vi "Configure Wavelength.vi"(7 "turret index (0)":u8, 8 "error in (no error)":errorcluster, 9 "reset (false)":bool, 10 "wavelength, nm":dbl, 11 "SOL MS in":refnum<class "PL SOL Instruments MS.lvclass">) -> (0 "error out":errorcluster, 1 "dispersion, nm/mm":dbl, 2 "wavelength, nm":dbl, 3 "SOL MS out":refnum<class "PL SOL Instruments MS.lvclass">)   [LabVIEW 2015, in "PL SOL Instruments MS.lvclass"]
doc: "Configures wavelength."
uses:
  PL SOL Instruments MS.lvclass
  PL SOL Instruments MS.lvclass/PL SOL Instruments MS.ctl
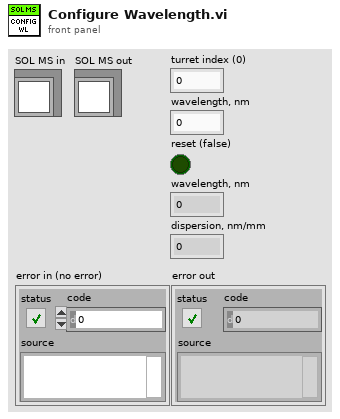
[diagram p1: front panel]
types:
  T1 = cluster{"name":string, "step timeout, ms":u32, "reset timeout, ms":u32, "gratings":cluster{"name":string, "step timeout, ms":u32, "reset timeout, ms":u32, "turret position":i32, "reset position":i32, "max position":i32, "backlash distance":i32, "step size, rad":dbl, "groove density, g/mm":dbl, "theta2, rad":dbl, "blaze wavelength, nm":dbl, "focal length, cm":dbl, "manual change":bool, "manual change position":i32}[], "current grating":cluster{"index":u8, "position":i32}}[]
  T2 = cluster{"name":string, "step timeout, ms":u32, "reset timeout, ms":u32, "gratings":cluster{"name":string, "step timeout, ms":u32, "reset timeout, ms":u32, "turret position":i32, "reset position":i32, "max position":i32, "backlash distance":i32, "step size, rad":dbl, "groove density, g/mm":dbl, "theta2, rad":dbl, "blaze wavelength, nm":dbl, "focal length, cm":dbl, "manual change":bool, "manual change position":i32}[], "current grating":cluster{"index":u8, "position":i32}}
  T3 = cluster{"name":string, "step timeout, ms":u32, "reset timeout, ms":u32, "turret position":i32, "reset position":i32, "max position":i32, "backlash distance":i32, "step size, rad":dbl, "groove density, g/mm":dbl, "theta2, rad":dbl, "blaze wavelength, nm":dbl, "focal length, cm":dbl, "manual change":bool, "manual change position":i32}[]
  T4 = cluster{"name":string, "step timeout, ms":u32, "reset timeout, ms":u32, "turret position":i32, "reset position":i32, "max position":i32, "backlash distance":i32, "step size, rad":dbl, "groove density, g/mm":dbl, "theta2, rad":dbl, "blaze wavelength, nm":dbl, "focal length, cm":dbl, "manual change":bool, "manual change position":i32}
  T5 = cluster{"turrets":cluster{"current grating index":u8, "wavelength, nm":dbl, "dispersion, nm/mm":dbl}[], "shutters":cluster{"is open":bool}[], "mirrors":cluster{"current position index":u8}[], "slits":cluster{"width, um":dbl}[]}
  T6 = cluster{"current grating index":u8, "wavelength, nm":dbl, "dispersion, nm/mm":dbl}[]
  T7 = cluster{"current grating index":u8, "wavelength, nm":dbl, "dispersion, nm/mm":dbl}
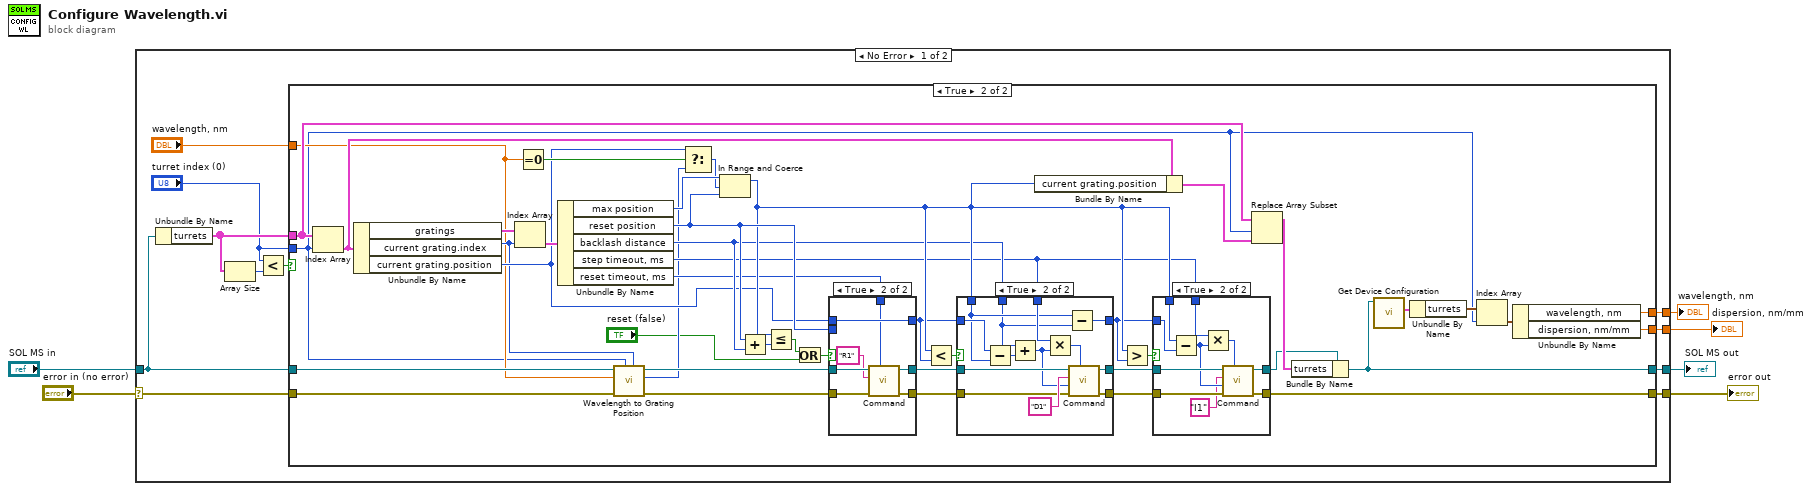
[diagram p0: block diagram]
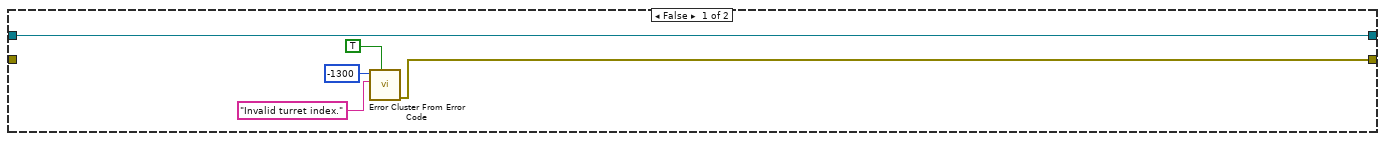
[diagram p2: hidden frame]
diagram:
  n1 = case shown="No Error" "error in (no error)" {
    selector: "error in (no error)" -> [w11 w105]
    tunnel: "SOL MS in" -> [w15 w104]
    tunnel: [w9 _] -> w5
    tunnel: [w8 _] -> w4
    tunnel: [w10 w105] -> w3
    tunnel: [w7 w104] -> w1
    frame No Error {
      n2 = Unbundle By Name(w15) -> ("turrets"=w17:T1)
      n3 = Array Size(array=w17) -> (size(s)=w14:i32)
      n4 = Less?(x="turret index (0)", y=w14) -> (x < y?=w12:bool)
      n5 = case shown="True" w12 {
        tunnel: w11 -> [_ w51]
        tunnel: w15 -> [w22 w49]
        tunnel: [w22 w41] -> w7
        tunnel: [w18 w61] -> w10
        tunnel: w17 -> [_ w59]
        tunnel: "wavelength, nm" -> [_ w47]
        tunnel: "turret index (0)" -> [_ w38]
        tunnel: [_ w40] -> w9
        tunnel: [_ w39] -> w8
        frame False {
          n6 = call <vilib>:"Error Cluster From Error Code.vi"("show call chain? (False)"=TRUE, "error message (\"\")"="Invalid turret index." ("error message (\"\")"), "error code (0)"=-1300) -> ("error out"=w18:errorcluster)  [unwired: 6 in]
        }
        frame True {
          n7 = Index Array(array=w59, index=w38) -> (element=w56:T2)
          n8 = Unbundle By Name(w56) -> ("gratings"=w58:T3, "current grating.index"=w48:u8, "current grating.position"=w53:i32)
          n9 = Index Array(array=w58, index=w48) -> (element=w57:T4)
          n10 = Equal To 0?(x=w47) -> (x = 0?=w54:bool)
          n11 = Unbundle By Name(w57) -> ("max position"=w65:i32, "reset position"=w64:i32, "backlash distance"=w62:i32, "step timeout, ms"=w60:u32, "reset timeout, ms"=w55:u32)
          n12 = call "Wavelength to Grating Position.vi"("grating index (0)"=w48, "turret index (0)"=w38, "error in (no error)"=w51, "wavelength, nm"=w47, "SOL MS in"=w49) -> ("error out"=w45:errorcluster, "grating position"=w46:i32, "SOL MS out"=w50:refnum<class "PL SOL Instruments MS.lvclass">)  [unwired: 4 in]
          n13 = Select(t=w53, s=w54, f=w46) -> (s? t:f=w52:i32)
          n14 = In Range and Coerce(upper limit=w65, x=w52, lower limit=w64) -> (coerced(x)=w63:i32)  [unwired: 1 out]
          n15 = Add(x=w64, y=w62) -> (x+y=w35:i32)
          n16 = Less Or Equal?(x=w63, y=w35) -> (x <= y?=w34:bool)
          n17 = Or(x=w34, y="reset (false)") -> (x .or. y?=w36:bool)
          n18 = case shown="True" w36 {
            tunnel: w50 -> [w96 w99]
            tunnel: w45 -> [w95 w100]
            tunnel: [w95 w101] -> w31
            tunnel: [w96 w102] -> w32
            tunnel: w53 -> [w94 _]
            tunnel: [w94 w103] -> w30
            tunnel: w64 -> [_ w103]
            tunnel: w55 -> [_ w97]
            frame False {
            }
            frame True {
              n19 = call "Command.vi"("additional timeout, ms (0)"=w97, "error in (no error)"=w100, "command"="R1", "SOL MS in"=w99) -> ("error out"=w101:errorcluster, "SOL MS out"=w102:refnum<class "PL SOL Instruments MS.lvclass">)  [unwired: 6 in]
            }
          }
          n20 = Less?(x=w63, y=w30) -> (x < y?=w33:bool)
          n21 = case shown="True" w33 {
            tunnel: w32 -> [w80 w87]
            tunnel: w31 -> [w79 w81]
            tunnel: [w79 w84] -> w29
            tunnel: [w80 w85] -> w28
            tunnel: w30 -> [w78 w91]
            tunnel: [w78 w90] -> w26
            tunnel: w63 -> [_ w89]
            tunnel: w62 -> [_ w88]
            tunnel: w60 -> [_ w92]
            frame False {
            }
            frame True {
              n22 = Subtract(x=w91, y=w89) -> (x-y=w93:i32)
              n23 = Add(x=w88, y=w93) -> (x+y=w82:i32)
              n24 = Multiply(x=w92, y=w82) -> (x*y=w86:u32)
              n25 = Subtract(x=w89, y=w88) -> (x-y=w90:i32)
              n26 = call "Command.vi"("additional timeout, ms (0)"=w86, "error in (no error)"=w81, "data"=w82, "command"="D1", "SOL MS in"=w87) -> ("error out"=w84:errorcluster, "SOL MS out"=w85:refnum<class "PL SOL Instruments MS.lvclass">)  [unwired: 5 in]
            }
          }
          n27 = Bundle By Name(cluster=w56, "current grating.position"=w63) -> (w25:T2)
          n28 = Greater?(x=w63, y=w26) -> (0:w27:bool)
          n29 = case shown="True" w27 {
            tunnel: w28 -> [w67 w73]
            tunnel: w29 -> [w66 w72]
            tunnel: [w66 w69] -> w61
            tunnel: [w67 w68] -> w23
            tunnel: w26 -> [_ w76]
            tunnel: w63 -> [_ w75]
            tunnel: w60 -> [_ w77]
            frame False {
            }
            frame True {
              n30 = Subtract(x=w75, y=w76) -> (x-y=w71:i32)
              n31 = Multiply(x=w77, y=w71) -> (x*y=w74:u32)
              n32 = call "Command.vi"("additional timeout, ms (0)"=w74, "error in (no error)"=w72, "data"=w71, "command"="I1", "SOL MS in"=w73) -> ("error out"=w69:errorcluster, "SOL MS out"=w68:refnum<class "PL SOL Instruments MS.lvclass">)  [unwired: 5 in]
            }
          }
          n33 = Replace Array Subset(array=w59, new element=w25, index=w38) -> (w24:T1)
          n34 = Bundle By Name(cluster=w23, "turrets"=w24) -> (w41:refnum<class "PL SOL Instruments MS.lvclass">)
          n35 = call "Get Device Configuration.vi"("SOL MS in"=w41) -> ("configuration"=w44:T5)  [unwired: 9 in, 1 out]
          n36 = Unbundle By Name(w44) -> ("turrets"=w43:T6)
          n37 = Index Array(array=w43, index=w38) -> (element=w42:T7)
          n38 = Unbundle By Name(w42) -> ("wavelength, nm"=w40:dbl, "dispersion, nm/mm"=w39:dbl)
        }
      }
    }
    frame Error {
    }
  }
  "wavelength, nm" <- w5
  "dispersion, nm/mm" <- w4
  "SOL MS out" <- w1
  "error out" <- w3
